vi "UE9 3-PWM Example.vi"(8 "error in":errorcluster, 9 "FIO0 Duty Cycle [%]":dbl=50.0 format="%.1f", 10 "16-bit PWM Frequency [Hz]":dbl=40.0 format="%.2f") -> (2 "Actual 16-bit Frequency":dbl format="%.1f")   [LabVIEW 2021]
panel:
  out "Update":bool
  out "Timer Value Array":u16[](array[numeric])
  in  "FIO2 Duty Cycle [%]":dbl=50.0 format="%.1f"
  in  "FIO1 Duty Cycle [%]":dbl=50.0 format="%.1f"
  in  "stop":bool
  out "Actual 8-bit Frequency":dbl format="%.1f"
  in  "FirstFound":bool=TRUE
  in  "Address":string="1"
  in  "ConnectionType":u16(ring) items=["LJ_ctUSB", "LJ_ctETHERNET"]
  out "TimerClockDivisor":u8
  out "TimerClockBase":dbl format="%.2f"
  out "Error Message":string
  # "Demonstrates 2 channels of 16-bit PWM output (FIO0 & FIO1) and 1 channel of 8-bit PWM output (FIO2).\nTimer clock, and timer clock divisor, are chosen to get as close as possible to the desired PWM frequency.\nFor 2.9<=f<=732.4, system clock is used for timer clock.\nFor f<2.9, fixed 750kHz timer clock is used for timer clock."
  # "This VI allows the duty cycles to\nbe changed while the VI is running."
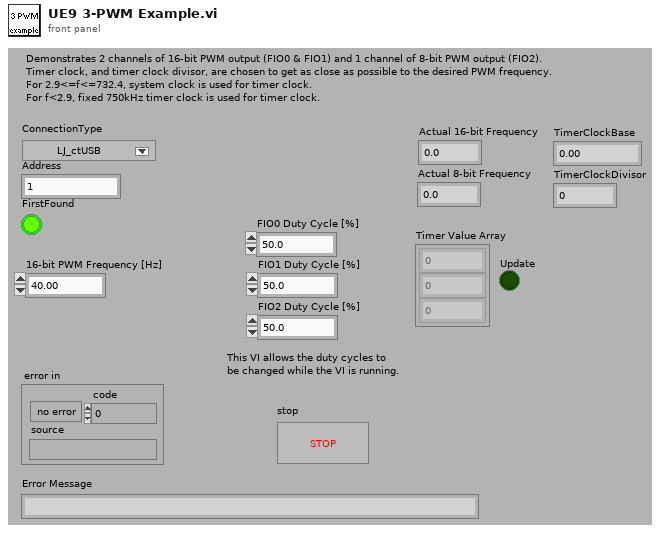
[diagram p1: front panel]
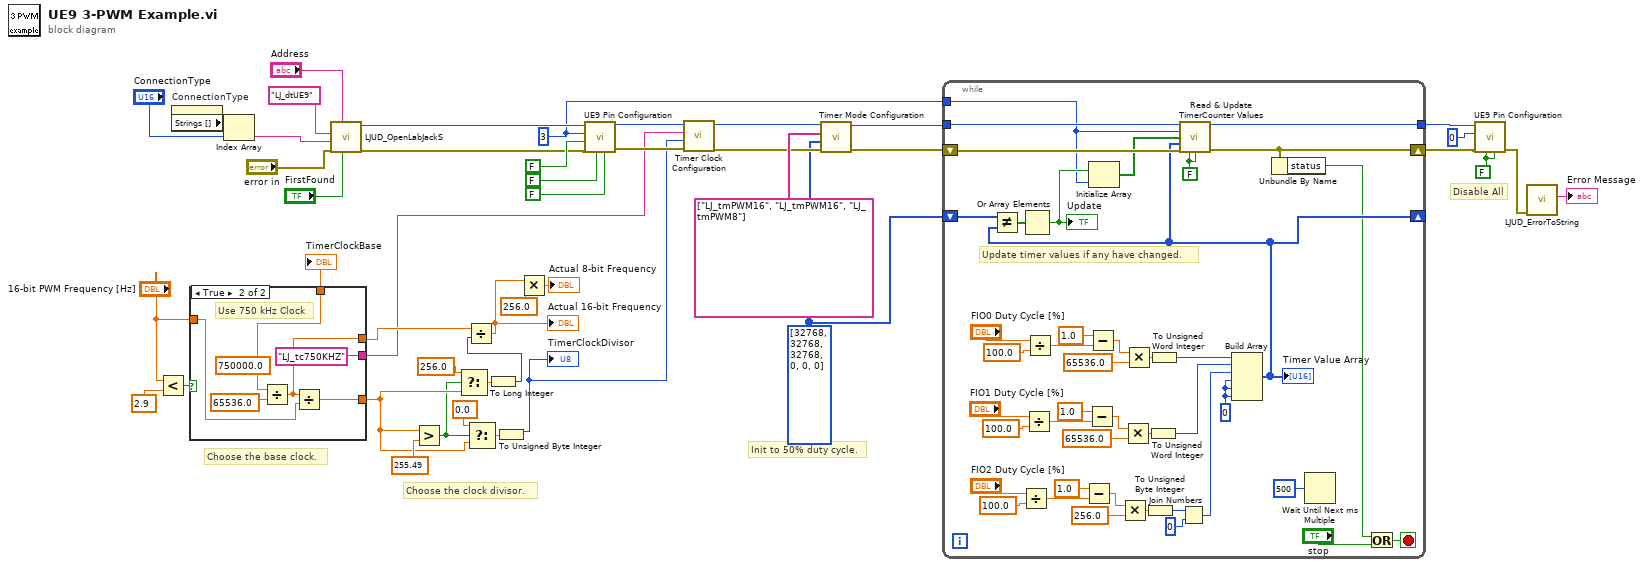
[diagram p0: block diagram]
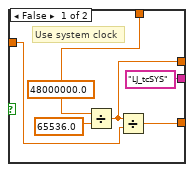
[diagram p2: hidden frame]
diagram:
  w1 = u8 3 ("Number of Timers Enabled")
  w25 = FALSE ("Enable Counter0")
  w2 = u16[] [32768, 32768, 32768, 0, 0, 0] ("TimerValues")
  # "Disable All"
  # "Choose the clock divisor."
  # "Choose the base clock."
  # "Init to 50% duty cycle."
  n1 = Less?(x="16-bit PWM Frequency [Hz]", y=2.9) -> (x < y?=w39:bool)
  n2 = property on="ConnectionType" class="Ring (strict)"() -> ("Strings []"=w19:string[])  [unwired: 2 in, 2 out]
  n3 = case shown="True" w39 {
    tunnel: "16-bit PWM Frequency [Hz]" -> [w50 w56]
    tunnel: [w49 w55] -> w33
    tunnel: [w47 w54] -> w29
    tunnel: [w48 w53] -> w30
    tunnel: ["LJ_tcSYS" ("Timer Clock Base") "LJ_tc750KHZ" ("Timer Clock Base")] -> w4
    frame False {
      w48 = 48000000.0 ("x")
      # "Use system clock"
      n4 = Divide(x=w48, y=65536.0) -> (x/y=w47:dbl)
      n5 = Divide(x=w47, y=w50) -> (x/y=w49:dbl)
    }
    frame True {
      w53 = 750000.0 ("x")
      # "Use 750 kHz Clock"
      n6 = Divide(x=w53, y=65536.0) -> (x/y=w54:dbl)
      n7 = Divide(x=w54, y=w56) -> (x/y=w55:dbl)
    }
  }
  "TimerClockBase" <- w30
  n8 = Index Array(array=w19, index="ConnectionType") -> (element=w17:string)
  n9 = call "LJUD_OpenLabJackS.vi"("FirstFound"="FirstFound", "Address"="Address", "error in"="error in", "ConnectionType"=w17, "DeviceType"="LJ_dtUE9") -> ("error out"=w5:errorcluster, "Handle"=w6:i32)  [unwired: 4 in, 1 out]
  n10 = Greater?(x=w33, y=255.49) -> (0:w32:bool)
  n11 = Select(t=256.0, s=w32, f=w33) -> (s? t:f=w35:dbl)
  n12 = Select(t=0.0, s=w32, f=w33) -> (s? t:f=w41:dbl)
  n13 = To Long Integer(number=w35) -> (32bit integer=w31:i32)
  n14 = Divide(x=w29, y=w31) -> (x/y=w28:dbl)
  "Actual 16-bit Frequency" <- w28
  n15 = To Unsigned Byte Integer(number=w41) -> (unsigned 8bit integer=w3:u8)
  "TimerClockDivisor" <- w3
  n16 = Multiply(x=w28, y=256.0) -> (x*y=→"Actual 8-bit Frequency":dbl)
  n17 = call "UE9 Pin Configuration.vi"("Enable Counter1"=FALSE ("Enable Counter0"), "Enable Counter0"=FALSE, "error in"=w5, "Enable DACs"=FALSE ("Enable Counter0"), "Number of Timers Enabled"=w1, "Handle In"=w6) -> ("error out"=w13:errorcluster, "Handle Out"=w12:i32)  [unwired: 4 in]
  n18 = call "Timer Clock Configuration.vi"("error in"=w13, "Timer Clock Divisor"=w3, "Timer Clock Base"=w4, "Handle In"=w12) -> ("error out"=w14:errorcluster, "Handle Out"=w11:i32)  [unwired: 6 in]
  n19 = call "Timer Mode Configuration.vi"("error in"=w14, "TimerValues"=w2, "TimerModes"=string[] ["LJ_tmPWM16", "LJ_tmPWM16", "LJ_tmPWM8"], "Handle In"=w11) -> ("error out"=w7:errorcluster, "Handle Out"=w8:i32)  [unwired: 6 in]
  n20 = while {
    shift-right: [w69] -> w22
    shift-left: w7 -> [w72]
    tunnel: w8 -> [w71]
    shift-right: [w63] -> _
    shift-left: w2 -> [w68]
    tunnel: [w64] -> w23
    tunnel: w1 -> [w59]
    stop <- w70 stop-if-true
    w58 = FALSE ("Reset Counter0")
    w73 = u16 0 ("PWM Timer Value")
    # "Update timer values if any have changed."
    n21 = Divide(x="FIO2 Duty Cycle [%]", y=100.0) -> (x/y=w97:dbl)
    n22 = Divide(x="FIO1 Duty Cycle [%]", y=100.0) -> (x/y=w87:dbl)
    n23 = Divide(x="FIO0 Duty Cycle [%]", y=100.0) -> (x/y=w82:dbl)
    n24 = Subtract(x=1.0, y=w97) -> (x-y=w95:dbl)
    n25 = Subtract(x=1.0, y=w87) -> (x-y=w89:dbl)
    n26 = Subtract(x=1.0, y=w82) -> (x-y=w80:dbl)
    n27 = Multiply(x=w95, y=256.0) -> (x*y=w92:dbl)
    n28 = Multiply(x=w89, y=65536.0) -> (x*y=w90:dbl)
    n29 = Multiply(x=w80, y=65536.0) -> (x*y=w79:dbl)
    n30 = To Unsigned Byte Integer(number=w92) -> (unsigned 8bit integer=w94:u8)
    n31 = To Unsigned Word Integer(number=w90) -> (unsigned 16bit integer=w75:u16)
    n32 = To Unsigned Word Integer(number=w79) -> (unsigned 16bit integer=w76:u16)
    n33 = Join Numbers(hi=w94, lo=u8 0) -> ((hi.lo)=w74:u16)
    n34 = Build Array(w76, w75, w74, w73, w73, w73) -> (w63:u16[])
    "Timer Value Array" <- w63
    n35 = Not Equal?(x=w68, y=w63) -> (x != y?=w67:bool[])
    n36 = Or Array Elements(Boolean array=w67) -> (logical OR=w66:bool)
    "Update" <- w66
    n37 = Initialize Array(w66, w59) -> (w65:bool[])
    n38 = call "Read & Update TimerCounter Values.vi"("Handle In"=w71, "# Timers to Read"=w59, "UpdateReset Timers"=w65, "TimerValues"=w63, "error in"=w72, "Read Counter0"=w58, "Read Counter1"=w58) -> ("Handle Out"=w64:i32, "error out"=w69:errorcluster)  [unwired: 5 in, 2 out]
    n39 = Unbundle By Name(w69) -> ("status"=w62:bool)
    n40 = Wait Until Next ms Multiple(millisecond multiple=u32 500) -> ()  [unwired: 1 out]
    n41 = Or(x=w62, y="stop") -> (x .or. y?=w70:bool)
  }
  n42 = call "UE9 Pin Configuration.vi"("Enable Counter1"=w25, "Enable Counter0"=w25, "error in"=w22, "Number of Timers Enabled"=u8 0 ("# Timers Enabled"), "Handle In"=w23) -> ("error out"=w21:errorcluster)  [unwired: 5 in, 1 out]
  n43 = call "LJUD_ErrorToString.vi"("error in"=w21) -> ("String"=→"Error Message":string)  [unwired: 10 in]
